vi "NewFolderDialog.vi"(8 "error in":errorcluster, 11 "ClassItemRefIn":refnum<vi>) -> (0 "error out":errorcluster, 1 "FolderNameOut":string="<class root>", 2 "FolderSourceScope":T1(ring), 3 "Cancelled":bool, 4 "FolderPath":path)   [LabVIEW 2020, in "ClassWriterNative.lvclass"]
uses:
  <resource>/Framework/Providers/Open_GDS/ClassProviders/Provider_LvNativeClass/ClassWriterNative_class/ClassWriterNative.lvclass
panel:
  in  "Visibility":T2(radio)
  in  "Type":enum32{"Virtual", "Real"}(radio)
  in  "Help":bool
  out "ProductPicture":picture
  in  "_ShowContextHelp":bool
  in  "New Folder Name":string caption="New Folder name"
  in  "_Cancel":bool
  in  "_Done":bool
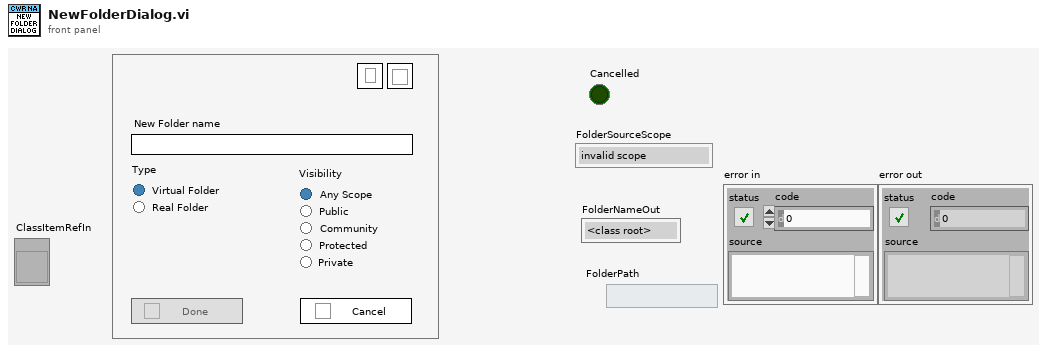
[diagram p1: front panel]
types:
  T1 = enum32{"invalid scope", "public", "private", "protected", "community"}
  T2 = enum32{"Any", "Public", "Community", "Protected", "Private"}
  T3 = cluster{"Cancelled":bool, "FolderSourceScope":enum32{"invalid scope", "public", "private", "protected", "community"}, "FolderNameOut":string, "FolderPath":path}
  T4 = enum32{"invalid scope", "public", "private", "protected", "community"}[]
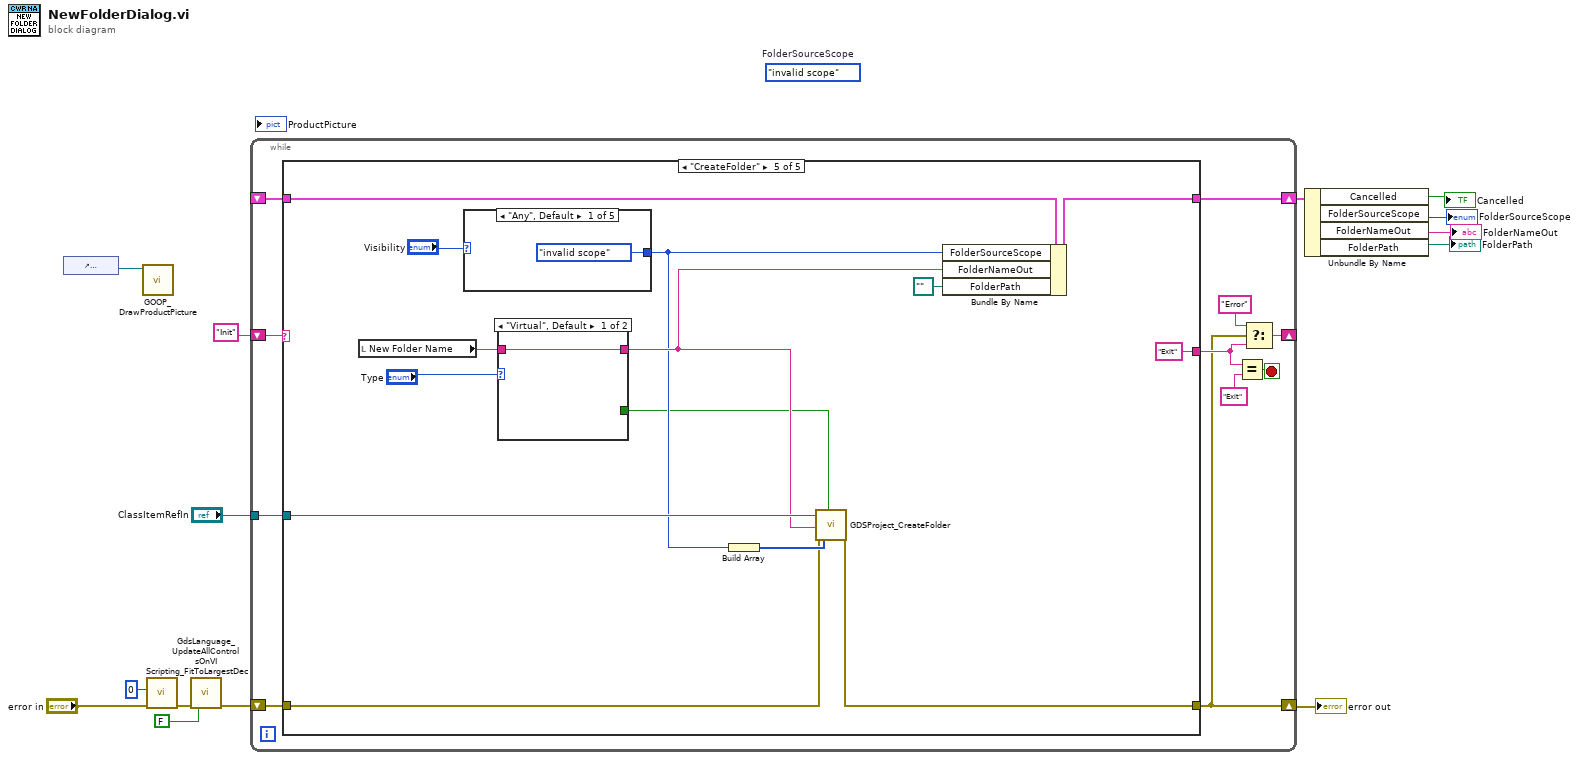
[diagram p0: block diagram]
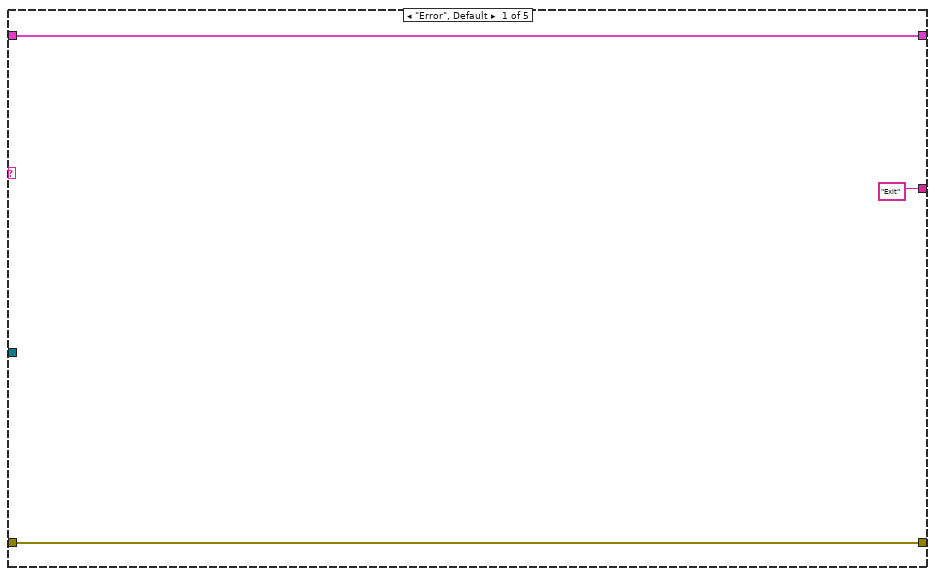
[diagram p2: hidden frame]
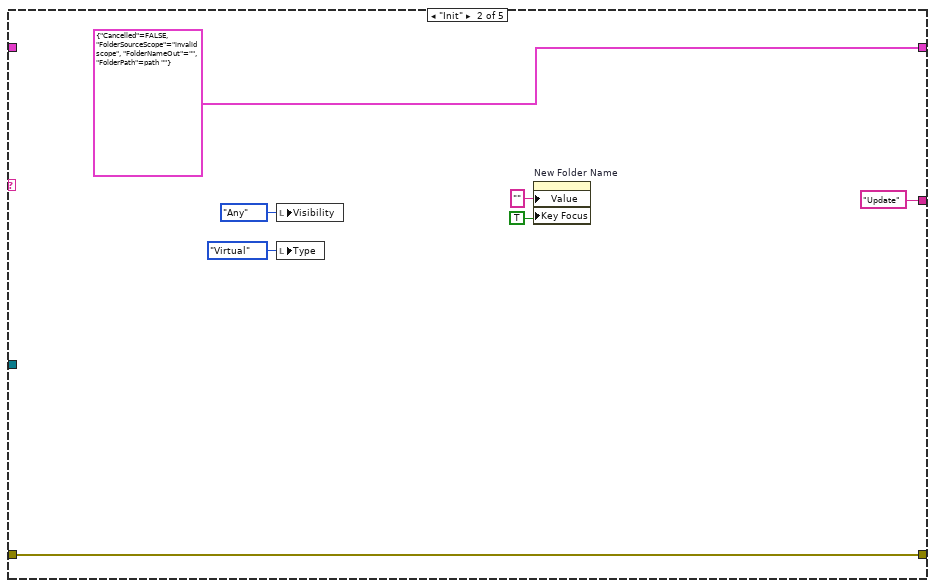
[diagram p3: hidden frame]
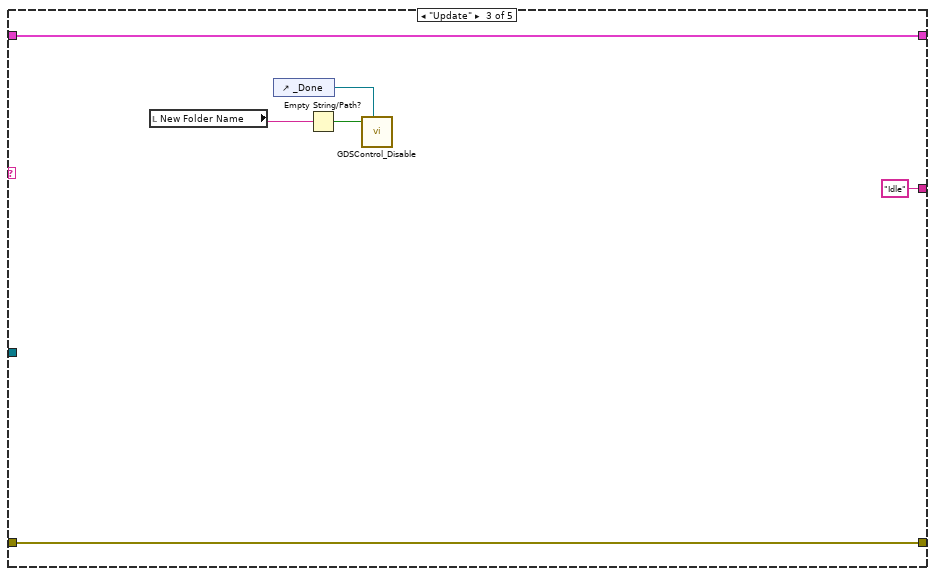
[diagram p4: hidden frame]
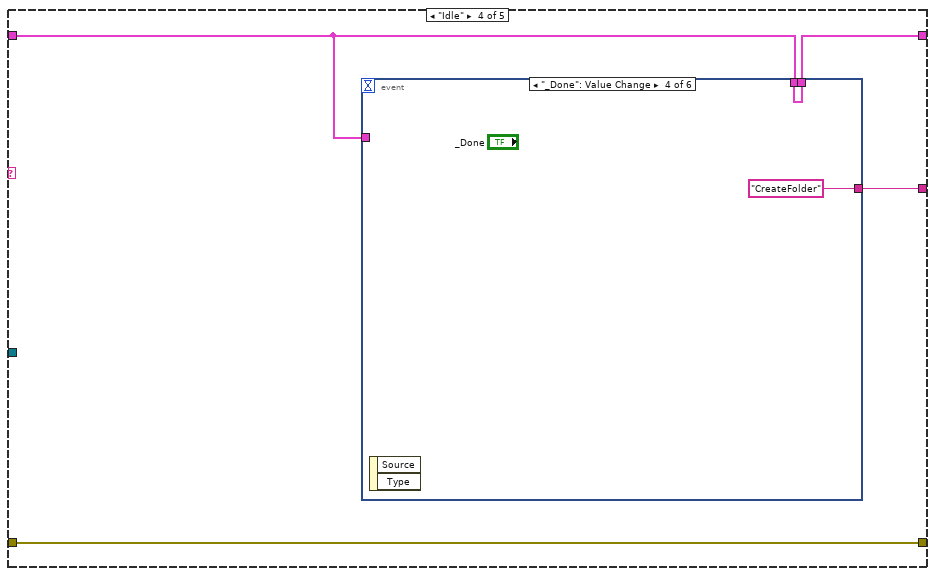
[diagram p5: hidden frame]
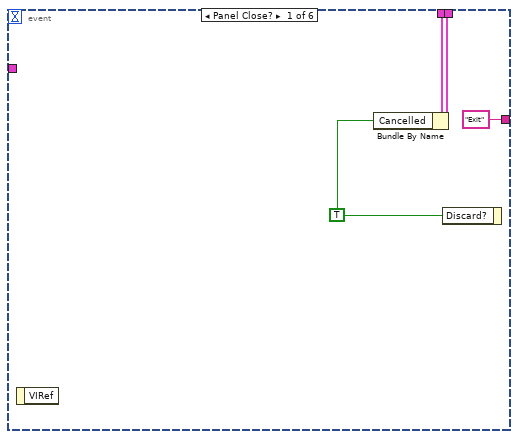
[diagram p6: hidden frame]
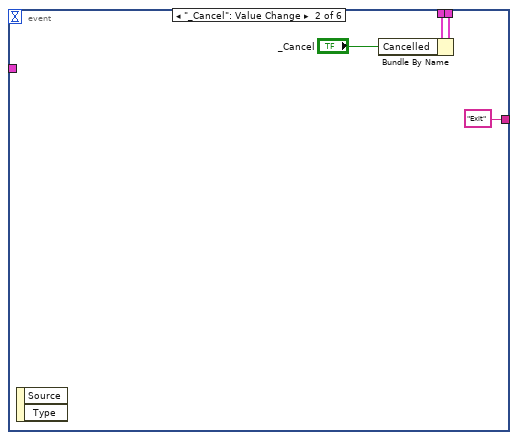
[diagram p7: hidden frame]
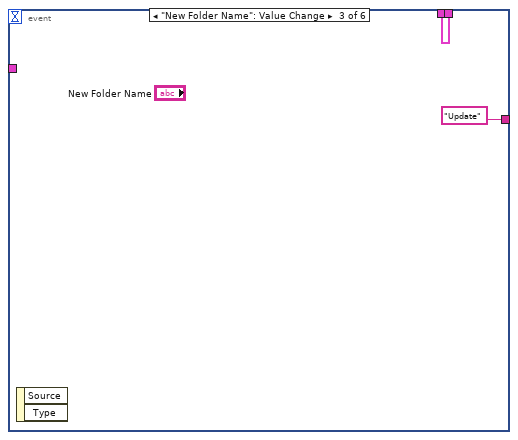
[diagram p8: hidden frame]
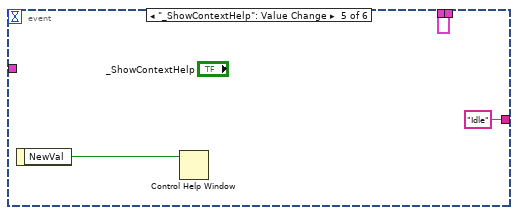
[diagram p9: hidden frame]
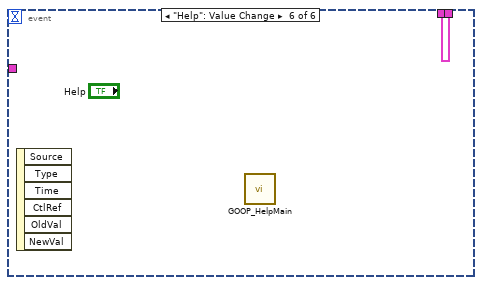
[diagram p10: hidden frame]
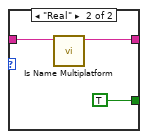
[diagram p11: hidden frame]
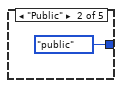
[diagram p12: hidden frame]
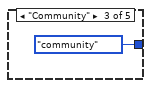
[diagram p13: hidden frame]
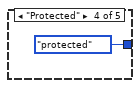
[diagram p14: hidden frame]
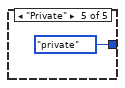
[diagram p15: hidden frame]
diagram:
  (unwired) T1."invalid scope"  # FolderSourceScope
  n1 = control-ref of="ProductPicture"() -> (w9:refnum<vi>)
  n2 = call <resource>:"GOOP_DrawProductPicture.vi"("ProductPictureControl"=w9) -> ()  [unwired: 10 in, 1 out]
  n3 = call <resource>:"Scripting_FitToLargestDec.vi"("error in (no error)"="error in", "border spacing (2 px)"=0) -> ("error out"=w7:errorcluster)  [unwired: 4 in, 1 out]
  n4 = call <resource>:"GdsLanguage_UpdateAllControlsOnVI.vi"("error in (no error)"=w7, "CreateLanguageFile(Use this to create a languageFile)"=FALSE) -> ("error out"=w11:errorcluster)  [unwired: 16 in, 1 out]
  n5 = while {
    shift-right: [w18] -> w1
    shift-left: w11 -> [w25]
    shift-right: [w23] -> _
    shift-left: "Init" -> [w24]
    shift-right: [w17] -> w13
    shift-left: _ -> [w16]
    tunnel: "ClassItemRefIn" -> [w15]
    stop <- w22 stop-if-true
    n6 = case shown="\"CreateFolder\"" w24 {
      tunnel: w25 -> [w28 w34 w39 w43 w62]
      tunnel: [w28 w34 w39 w43 w63] -> w18
      tunnel: ["Exit" "Update" "Idle" w44 "Exit"] -> w19
      tunnel: [w26 T3 {"Cancelled"=FALSE, "FolderSourceScope"=enum."invalid scope", "FolderNameOut"="", "FolderPath"=path ""} w40 w45 w73] -> w17
      tunnel: w16 -> [w26 _ w40 w42 w75]
      tunnel: w15 -> [_ _ _ _ w68]
      frame "Error", Default {
      }
      frame "Init" {
        n7 = local write "Visibility"(T2."Any" ("Visibility")) -> ()
        n8 = local write "Type"(enum32{"Virtual", "Real"}."Virtual" ("Type")) -> ()
        n9 = property on="New Folder Name" class="Str"("Value"="" ("New Folder Name"), "Key Focus"=TRUE) -> ()  [unwired: 2 in, 2 out]
      }
      frame "Update" {
        n10 = local read "New Folder Name"() -> (w38:string)
        n11 = control-ref of="_Done"() -> (w36:refnum<vi>)
        n12 = Empty String/Path?(string/path=w38) -> (empty?=w37:bool)
        n13 = call <resource>:"GDSControl_Disable.vi"("ControlRefnum(IgnoreIfNotWired)"=w36, "Disasble(True)"=w37) -> ()  [unwired: 9 in, 1 out]
      }
      frame "Idle" {
        n14 = event shown="[3] \"_Done\": Value Change" {
          selector: _ -> [_ _ _ _ _ _]
          dyn-events: _ -> [_ _ _ _ _ _]
          timeout: _ -> [_ _ _ _ _ _]
          tunnel: w42 -> [w48 w53 w55 w57 w60 w61]
          tunnel: [w47 w52 w55 w57 w60 w61] -> w45
          tunnel: ["Exit" "Exit" "Update" "CreateFolder" "Idle" _] -> w44
          tunnel: w42 -> [_ _ _ _ _ _]
          event Panel Close? {
            w46 = TRUE ("Discard?")
            n15 = event-data() -> ()  [unwired: 1 in, 1 out]
            n16 = Bundle By Name(cluster=w48, "Cancelled"=w46) -> (w47:T3)
            n17 = event-data("Discard?"=w46) -> ()  [unwired: 1 in, 1 out]
          }
          event "_Cancel": Value Change {
            n18 = event-data() -> ()  [unwired: 1 in, 2 out]
            n19 = Bundle By Name(cluster=w53, "Cancelled"="_Cancel") -> (w52:T3)
          }
          event "New Folder Name": Value Change {
            n20 = event-data() -> ()  [unwired: 1 in, 2 out]
          }
          event "_Done": Value Change {
            n21 = event-data() -> ()  [unwired: 1 in, 2 out]
          }
          event "_ShowContextHelp": Value Change {
            n22 = event-data() -> ("NewVal"=w58:bool)  [unwired: 1 in]
            n23 = Control Help Window(1:w58) -> ()  [unwired: 1 in]
          }
          event "Help": Value Change {
            n24 = event-data() -> ()  [unwired: 1 in, 6 out]
            n25 = call <resource>:"GOOP_HelpMain.vi"() -> ()  [unwired: 12 in]
          }
        }
      }
      frame "CreateFolder" {
        n26 = local read "New Folder Name"() -> (w70:string)
        n27 = case shown="\"Any\", Default" "Visibility" {
          tunnel: [T1."invalid scope" ("FolderSourceScope") T1."public" ("FolderSourceScope") T1."community" ("FolderSourceScope") T1."protected" ("FolderSourceScope") T1."private" ("FolderSourceScope")] -> w66
          frame "Any", Default {
          }
          frame "Public" {
          }
          frame "Community" {
          }
          frame "Protected" {
          }
          frame "Private" {
          }
        }
        n28 = case shown="\"Virtual\", Default" "Type" {
          tunnel: w70 -> [w76 w79]
          tunnel: [w76 w78] -> w67
          tunnel: [_ TRUE] -> w64
          frame "Virtual", Default {
          }
          frame "Real" {
            n29 = call <vilib>:"Is Name Multiplatform.vi"("filename"=w79) -> ("suggested filename"=w78:string)  [unwired: 6 in, 4 out]
          }
        }
        n30 = Build Array(w66) -> (w65:T4)
        n31 = call <resource>:"GDSProject_CreateFolder.vi"("Project Item To Create Folder Below(Use MyComputer if not wired)"=w68, "FolderName"=w67, "error in (no error)"=w62, "FolderScope"=w65, "CreateThePhysicalFolderIfPossible(False)"=w64) -> ("error out"=w63:errorcluster)  [unwired: 11 in, 3 out]
        n32 = Bundle By Name(cluster=w75, "FolderSourceScope"=w66, "FolderNameOut"=w67, "FolderPath"=path "") -> (w73:T3)
      }
    }
    n33 = Equal?(x=w19, y="Exit") -> (x = y?=w22:bool)
    n34 = Select(t="Error", s=w18, f=w19) -> (s? t:f=w23:string)
  }
  "error out" <- w1
  n35 = Unbundle By Name(w13) -> ("Cancelled"=→"Cancelled":bool, "FolderSourceScope"=→"FolderSourceScope":T1, "FolderNameOut"=→"FolderNameOut":string, "FolderPath"=→"FolderPath":path)
